vi "temp_condition.vi"() -> ()   [LabVIEW 2023]
panel:
  out "Temperature Condition":string
  in  "Knob":dbl(knob) scale=0.0..50.0
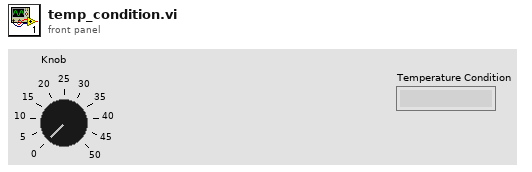
[diagram p1: front panel]
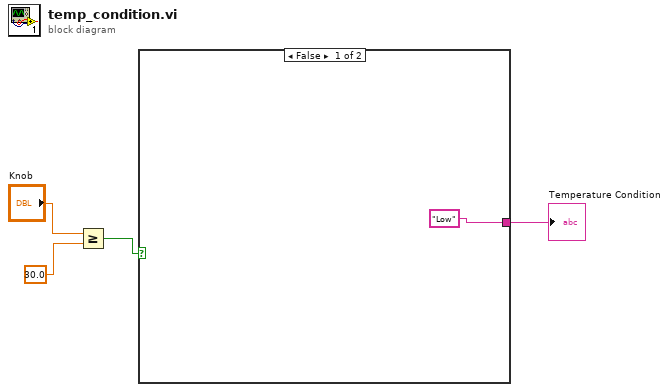
[diagram p0: block diagram]
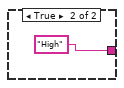
[diagram p2: hidden frame]
diagram:
  n1 = Greater Or Equal?(x="Knob", y=30.0) -> (x >= y?=w2:bool)
  n2 = case shown="False" w2 {
    tunnel: ["Low" "High"] -> w4
    frame False {
    }
    frame True {
    }
  }
  "Temperature Condition" <- w4
